vi "Format Timestamp Into String (ms resolution).vi"(1 "Timestamp":timestamp) -> (0 "Timestamp String (ms resolution)":string)   [LabVIEW 2016, in "Error Manager.lvlib"]
doc: "This VI converts a timestamp into a string such as 2023-09-01 15:10:17.520"
uses:
  Error Manager.lvlib
panel:
  # "Development\nControls or indicators that are useful for development or testing, but which are not outputs of the VI."
  # "Input\nInputs to the VI"
  # "Output\nOutputs of the VI"
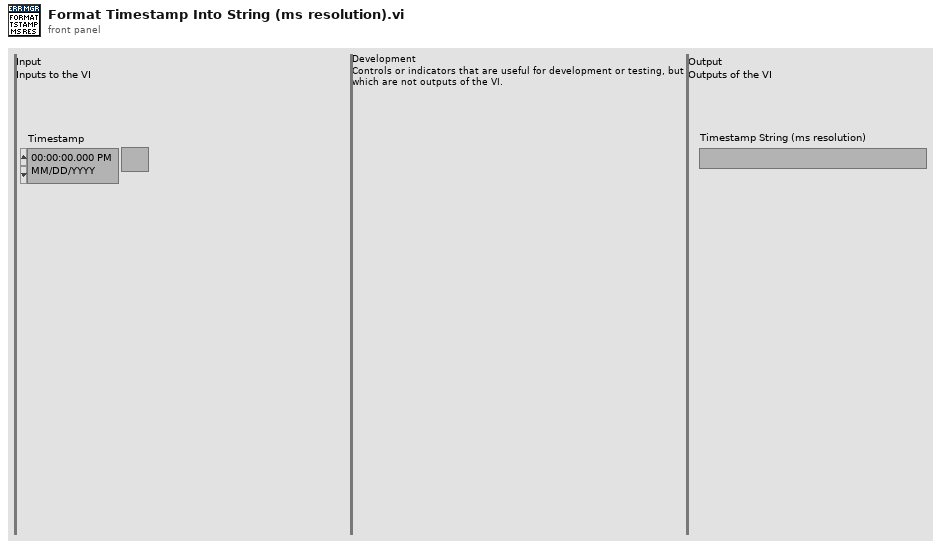
[diagram p1: front panel]
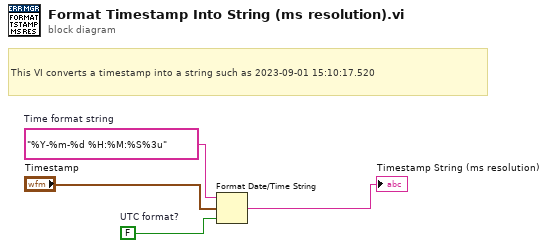
[diagram p0: block diagram]
diagram:
  w3 = FALSE  # UTC format?
  w4 = "%Y-%m-%d %H:%M:%S%3u"  # Time format string
  # "This VI converts a timestamp into a string such as 2023-09-01 15:10:17.520"
  n1 = Format Date/Time String(time format string (%c)=w4, seconds (now)="Timestamp", UTC format=w3) -> (date/time string=→"Timestamp String (ms resolution)":string)
